vi "to string.vi"(8 "error in":errorcluster, 11 "SystemLin Tag Module configuration in":refnum<class "SystemLink configuration.lvclass">) -> (0 "error out":errorcluster, 1 "data":string, 2 "version":string, 3 "SystemLin Tag Module configuration out":refnum<class "SystemLink configuration.lvclass">)   [LabVIEW 2015, in "SystemLink configuration.lvclass"]
doc: "Provides an interface for saving a module configuration to a file or other serialized data source. It is recommended that all children of this class store data in two sets--data required for its own initialization, and any data required for parent initialization--and that each implementation uses the <b>Call Parent Method</b> primitive to serialize parent information."
uses:
  SystemLink configuration.lvclass
  SystemLink configuration.lvclass/SystemLink configuration.ctl
  current version.vi
  <vilib>/NI/Tag Bus Module Framework/module configuration/TBM module configuration.lvclass
  <vilib>/NI/Tag Bus Module Framework/channel/TBM channel.lvclass
  <vilib>/NI/Configuration Framework/serializable configuration/NISE_CEF_serializable configuration.lvclass
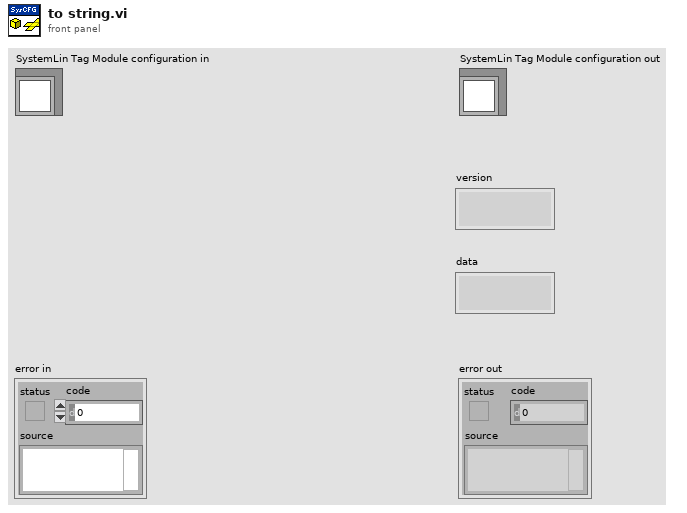
[diagram p1: front panel]
types:
  T1 = typedef "SystemLink configuration.lvclass/Line.ctl" = cluster{"channel":refnum<class "TBM channel.lvclass">, "Data Tag Type":T2}
  T2 = typedef "SystemLink configuration.lvclass/Data Tag Type.ctl" = enum16{"Double", "Single", "I32", "I16", "I8", "U64", "U32", "U16", "U8", "Boolean", "String", "Timestamp"}
  T3 = typedef "SystemLink configuration.lvclass/Connection Configuration.ctl" = cluster{"Connection Type":T4, "AMQP":cluster{"Configuration ID":string}, "HTTP":cluster{"Verify Server?":bool, "Server URL":string, "CA Certificate File":string, "User Info":cluster{"Username":string, "Password":string}, "API Key":string}}
  T4 = typedef "SystemLink configuration.lvclass/Connection Type.ctl" = enum16{"AMQP", "HTTP", "API Key (SystemLink Cloud)"}
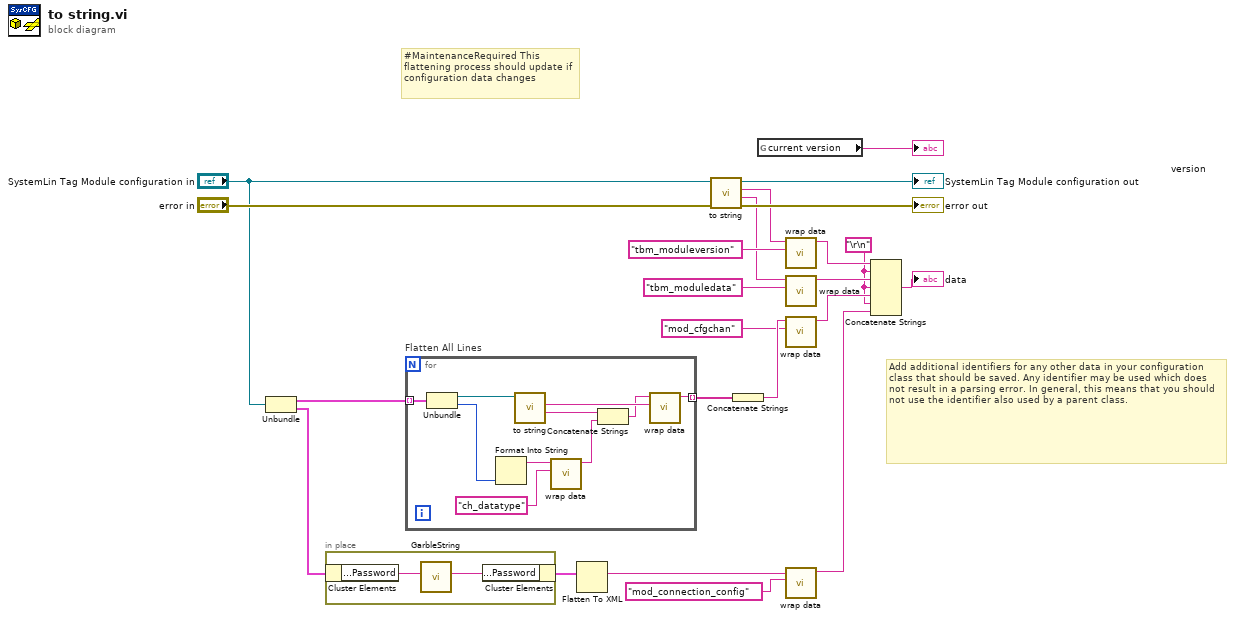
[diagram p0: block diagram]
diagram:
  w6 = "\r\n"
  # "Add additional identifiers for any other data in your configuration class that should be saved. Any identifier may be used which does not result in a parsing error. In general, this means that you should not use the identifier also used by a parent class."
  # "#MaintenanceRequired This flattening process should update if configuration data changes"
  n1 = Unbundle("SystemLin Tag Module configuration in") -> (w10:T1[], w2:T3)
  n2 = in-place {
    n3 = in-place-cluster #1(w2) -> ("HTTP.User Info.Password"=w25:string)
    n4 = call "GarbleString.vi"("String In"=w25) -> ("String Out"=w24:string)  [unwired: 10 in]
    n5 = in-place-cluster #1("HTTP.User Info.Password"=w24) -> (w1:T3)
  }
  n6 = for "Flatten All Lines" {
    tunnel: w10 -> [w35] mode=indexing
    tunnel: [w28] -> w9 mode=indexing
    n7 = Unbundle(w35) -> ("channel"=w34:refnum<class "TBM channel.lvclass">, "Data Tag Type"=w31:T2)
    n8 = Format Into String(w31) -> (resulting string=w30:string)  [unwired: 3 in, 1 out]
    n9 = call-dynamic "to string.vi"("channel in"=w34) -> ("channel data"=w32:string, "identifier"=w33:string)  [unwired: 7 in, 2 out]
    n10 = call <vilib>:"wrap data.vi"("identifier"="ch_datatype", "data to wrap"=w30) -> ("wrapped data"=w26:string)  [unwired: 9 in]
    n11 = Concatenate Strings(w32, w26) -> (w27:string)
    n12 = call <vilib>:"wrap data.vi"("identifier"=w33, "data to wrap"=w27) -> ("wrapped data"=w28:string)  [unwired: 9 in]
  }
  n13 = Flatten To XML(anything=w1) -> (xml string=w5:string)
  n14 = call-parent "to string.vi"("error in"="error in", "module configuration in"="SystemLin Tag Module configuration in") -> ("error out"=→"error out":errorcluster, "data"=w14:string, "version"=w15:string, "module configuration out"=→"SystemLin Tag Module configuration out":refnum<class "SystemLink configuration.lvclass">)  [unwired: 6 in]
  n15 = Concatenate Strings(w9) -> (w8:string)
  n16 = global read "current version.vi" "current version"() -> (→"version":string)
  n17 = call <vilib>:"wrap data.vi"("identifier"="tbm_moduleversion" ("additional identifier"), "data to wrap"=w15) -> ("wrapped data"=w17:string)  [unwired: 9 in]
  n18 = call <vilib>:"wrap data.vi"("identifier"="tbm_moduledata" ("additional identifier"), "data to wrap"=w14) -> ("wrapped data"=w16:string)  [unwired: 9 in]
  n19 = call <vilib>:"wrap data.vi"("identifier"="mod_cfgchan", "data to wrap"=w8) -> ("wrapped data"=w11:string)  [unwired: 9 in]
  n20 = call <vilib>:"wrap data.vi"("identifier"="mod_connection_config", "data to wrap"=w5) -> ("wrapped data"=w4:string)  [unwired: 9 in]
  n21 = Concatenate Strings(w17, w6, w16, w6, w11, w6, w4) -> (→"data":string)
